vi "报告-报警采集.vi"   [LabVIEW 2015]
uses:
  Global control/global-1.vi
  Global control/global-Report.vi
  Global control/global-2.vi
  Global control/global-opc.vi
types:
  T1 = cluster{"Host交流故障":bool, "Host交流缺相":bool, "Host交流失电":bool, "01#JLCL交流故障":bool, "01#JLCL交流缺相":bool, "01#JLCL交流失电":bool, "02#JLCL交流故障":bool, "02#JLCL交流缺相":bool, "02#JLCL交流失电":bool, "备用1":bool, "备用2":bool, "备用3":bool, "备用4":bool, "备用5":bool, "备用6":bool, " 备用7":bool}
  T2 = cluster{"09#电源模块故障":bool, "10#电源模块故障":bool, "11#电源模块故障":bool, "12#电源模块故障":bool, "13#电源模块故障":bool, "14#电源模块故障":bool, "15#电源模块故障":bool, "16#电源模块故障":bool, "01#电源模块故障":bool, "02#电源模块故障":bool, "03#电源模块故障":bool, "04#电源模块故障":bool, "05#电源模块故障":bool, "06#电源模块故障":bool, "07#电源模块故障":bool, " 08#电源模块故障":bool}
  T3 = cluster{"09#模块通信故障":bool, "10#模块通信故障":bool, "11#模块通信故障":bool, "12#模块通信故障":bool, "13#模块通信故障":bool, "14#模块通信故障":bool, "15#模块通信故障":bool, "16#模块通信故障":bool, "01#模块通信故障":bool, "02#模块通信故障":bool, "03#模块通信故障":bool, "04#模块通信故障":bool, "05#模块通信故障":bool, "06#模块通信故障":bool, "07#模块通信故障":bool, "08#模块通信故障":bool}
  T4 = cluster{"母线过压":bool, "母线欠压":bool, "母线绝缘异常":bool, "母线绝缘预警":bool, "母线绝缘压差故障":bool, "母线交流串入故障":bool, "备用5":bool, " 备用6":bool, "电池组过压":bool, "电池组欠压":bool, "电池组过温":bool, "单体电池故障":bool, "备用1":bool, "备用2":bool, "备用3":bool, " 备用4":bool}
  T5 = cluster{"合母输出3#告警":bool, "合母输出4#告警":bool, "合母输出5#告警":bool, "合母输出6#告警":bool, "13#开关状态":bool, "14#开关状态":bool, "15#开关状态":bool, "16#开关状态":bool, "控母输出1#告警":bool, "控母输出2#告警":bool, "控母输出3#告警":bool, "控母输出4#告警":bool, "控母输出5#告警":bool, "控母输出6#告警":bool, "合母输出1#告警":bool, "合母输出2#告警":bool}
  T6 = cluster{"动作报告1":bool, "动作报告2":bool, "动作报告3":bool, "动作报告4":bool, "动作报告5":bool, "动作报告6":bool, "动作报告7":bool, "动作报告8":bool, "动作报告9":bool, "动作报告10":bool, "动作报告11":bool, "动作报告12":bool, "动作报告13":bool, "动作报告14":bool, "动作报告15":bool, "动作报告16":bool, "重合闸成功":bool, "线路测试失败":bool, "重合闸失败":bool, "手动合闸失败":bool, "一次重合":bool, "二次重合":bool, "三次重合":bool, "四次重合":bool, "失灵保护跳闸":bool, "失灵保护重跳":bool}
  T7 = cluster{"动作信号":bool, "异常告警":bool, "断路器合闸位置":bool, "隔离开关合闸位置":bool, "远方就地（1就地）":bool, "扩展板异常告警":bool, "虚遥信7":bool, "虚遥信8":bool, "虚遥信9":bool, "虚遥信10":bool, "虚遥信11":bool, "虚遥信12":bool, "虚遥信13":bool, "虚遥信14":bool, "虚遥信15":bool, "虚遥信16":bool}
  T8 = cluster{"直接合闸":bool, "分闸复位":bool, "带测合闸":bool, "MCB故障":bool, "断路器合闸反馈信号":bool, "ED储能":bool, "应急分闸":bool, "断路器分闸反馈信号":bool, "远程控制":bool, "就地控制":bool, "试验位置":bool, "工作位置":bool, "带测接触器":bool, "本站框架":bool, "邻站过流":bool, "邻站框架":bool}
  T9 = cluster{"toHMI正常运行":bool, "toHMI异常跳闸":bool, "toHMI远程":bool, "toHMI模拟中压合闸—按钮":bool, "toHMI负极柜故障报警":bool, "toHMI正极柜故障报警":bool, "toHMI馈线柜故障报警":bool, "toHMI上网柜故障报警":bool, "toHMI整流柜故障报警":bool, "toHMI压敏快熔故障":bool, "toHMI整流柜跳闸":bool, "toHMI整流柜合闸—状态":bool, "直流电流输出":u32, "直流220V电压输出":u32, "380电压输入":u32, "模拟中压合闸控制":bool, "toHMI本地":bool}
  T10 = cluster{"toHMI正常运行":bool, "toHMI设备准备好":bool, "toHMI设备异常":bool, "toHMI刀开关合—状态":bool, "toHMI刀开关分—状态":bool, "toHMI刀开关合按钮":bool, "toHMI刀开关分按钮":bool, "toHMI复位按钮":bool, "toHMI远程":bool, "toHMI本地":bool, "toHMI刀闸合—动作":bool, "toHMI刀闸分—动作":bool, "刀开关合闸控制":bool, "刀开关分闸控制":bool, "故障复位控制":bool}
  T11 = cluster{"toHMI正常运行":bool, "toHMI设备准备好":bool, "toHMI设备异常":bool, "toHMI高断分—状态":bool, "toHMI高断合—状态":bool, "toHMI继保故障信号":bool, "toHMI远方":bool, "toHMI本地":bool, "toHMI旁路合闸—按钮":bool, "toHMI旁路分闸—按钮":bool, "toHMI允许高断合闸—状态":bool, "toHMI旁路合分闸—状态":bool, "1500V电压输出":u32, "高断储能控制":bool, "旁路合闸控制":bool, "旁路分闸控制":bool}
  T12 = cluster{"toHMI正常运行":bool, "toHMI设备准备好":bool, "toHMI设备异常":bool, "toHMI刀开关分—状态":bool, "toHMI刀开关合—状态":bool, "toHMI框架电流故障":bool, "toHMI框架电压故障":bool, "toHMII段电压故障":bool, "toHMIII段电压故障":bool, "toHMI装置故障":bool, "toHMIMCB故障":bool, "toHMI刀开关合—完成":bool, "toHMI复位按钮":bool, "toHMI远程":bool, "toHMI本地":bool, "模拟电流框架故障控制":bool, "模拟电压框架故障控制":bool, "模拟I段电压故障控制":bool, "模拟II段电压故障控制":bool, "故障复位控制":bool}
  T13 = cluster{"toHMI刀开关合—状态":bool, "toHMI刀开关分—状态":bool, "toHMI刀开关合按钮":bool, "toHMI刀开关分按钮":bool, "toHMI远程":bool, "toHMI本地":bool, "toHMI正常运行":bool, "toHMI设备准备好":bool, "toHMI设备异常":bool, "toHMI刀闸合—动作":bool, "toHMI刀闸分—动作":bool, "toHMI接触轨有压":bool, "刀开关合闸控制":bool, "刀开关分闸控制":bool}
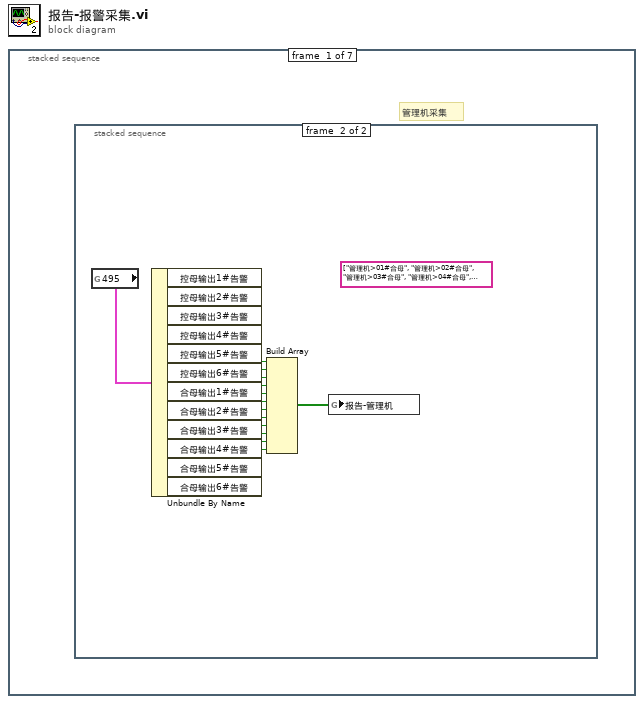
[diagram p0: block diagram]
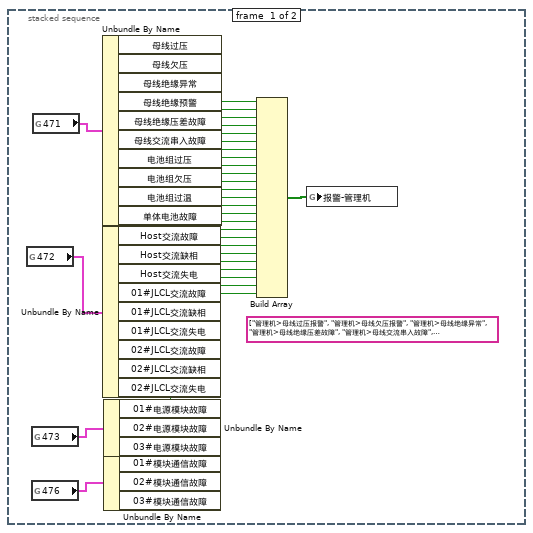
[diagram p2: hidden frame]
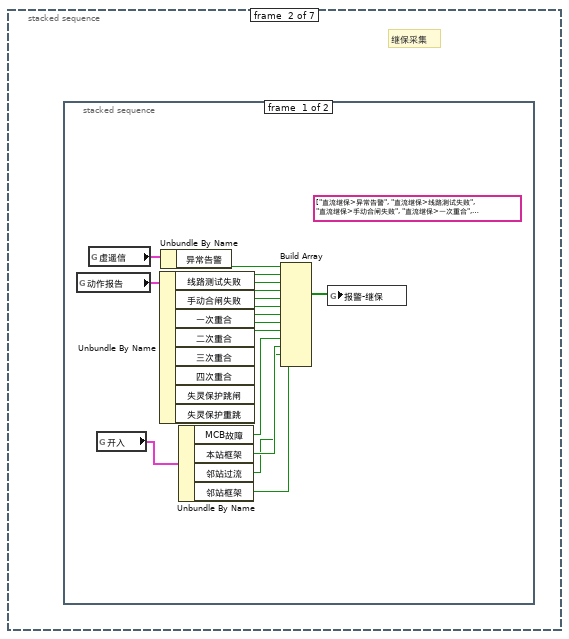
[diagram p3: hidden frame]
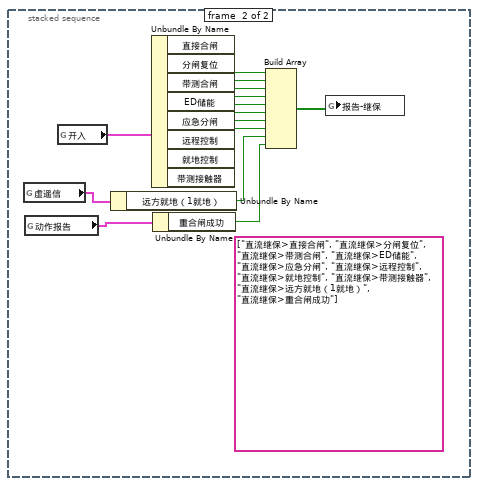
[diagram p4: hidden frame]
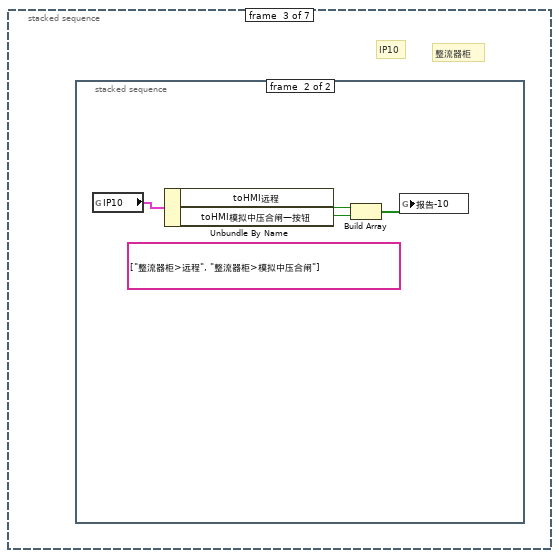
[diagram p5: hidden frame]
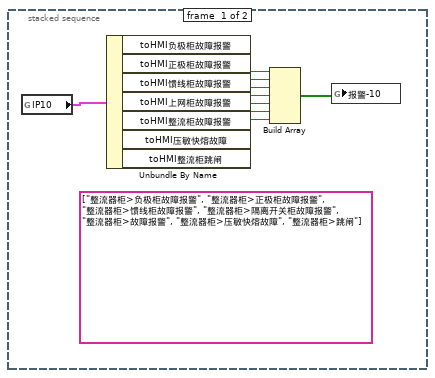
[diagram p6: hidden frame]
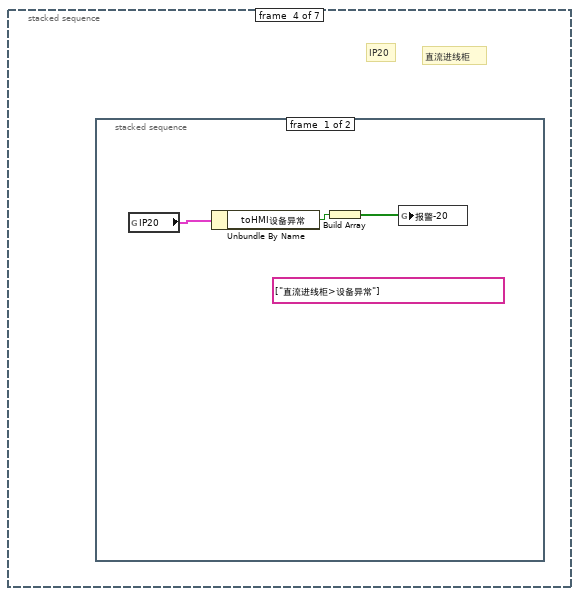
[diagram p7: hidden frame]
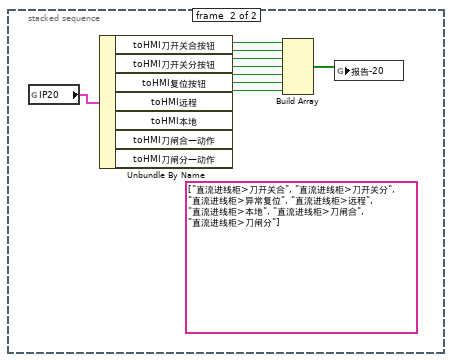
[diagram p8: hidden frame]
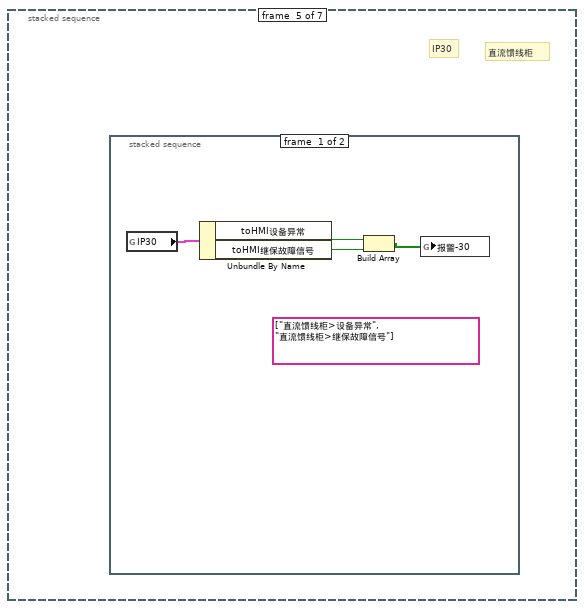
[diagram p9: hidden frame]
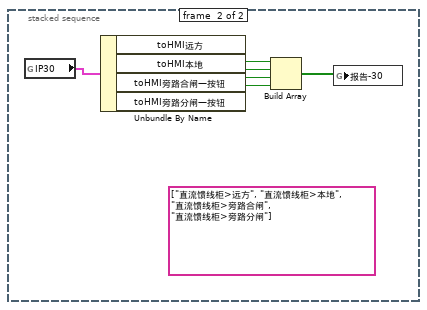
[diagram p10: hidden frame]
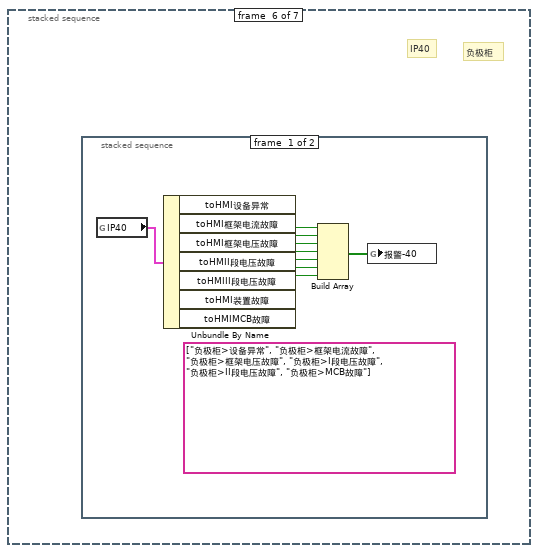
[diagram p11: hidden frame]
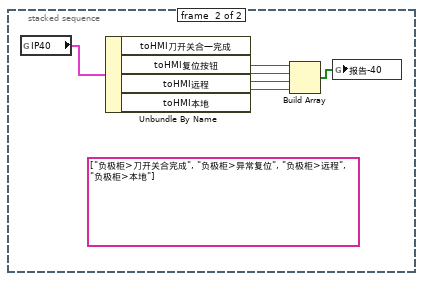
[diagram p12: hidden frame]
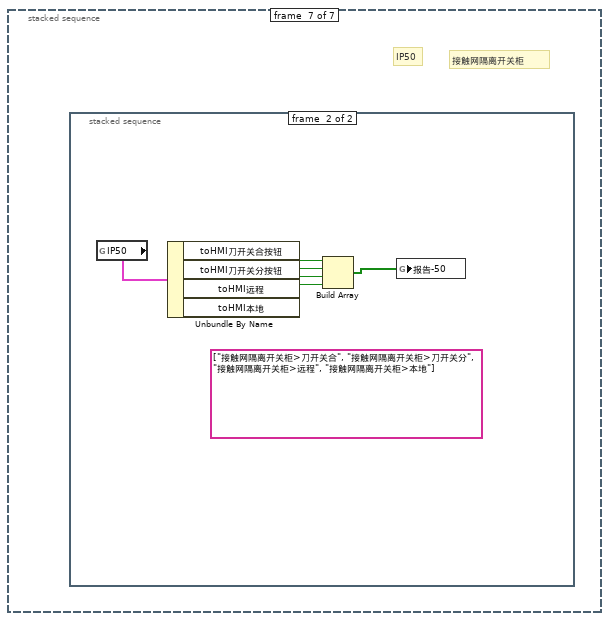
[diagram p13: hidden frame]
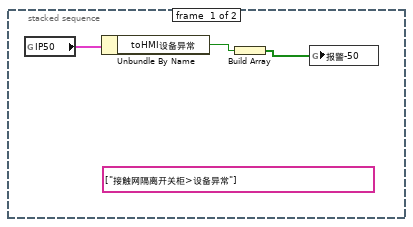
[diagram p14: hidden frame]
diagram:
  n1 = stacked-sequence {
    frame #0 {
      # "管理机采集"
      n2 = stacked-sequence {
        frame #0 {
          (unwired) string[] ["管理机>母线过压报警", "管理机>母线欠压报警", "管理机>母线绝缘异常", "管理机>母线绝缘压差故障", "管理机>母线交流串入故障", "管理机>电池组过压", "管理机>电池组欠压", "管理机>电池组过温", "管理机>单体电池故障", "管理机>Host交流故障", "管理机>Host交流缺相", "管理机>Host交流失电", "管理机>01#JLCL交流故障", "管理机>01#JLCL交流缺相", "管理机>01#JLCL交流失电", "管理机>02#JLCL交流故障", "管理机>02#JLCL交流缺相", "管理机>02#JLCL交流失电", "管理机>01#电源模块故障", "管理机>02#电源模块故障", "管理机>03#电源模块故障", "管理机>01##模块通信故障", "管理机>02##模块通信故障", "管理机>03##模块通信故障"]
          n3 = global read "global-1.vi" "472"() -> (w29:T1)
          n4 = global read "global-1.vi" "473"() -> (w28:T2)
          n5 = global read "global-1.vi" "476"() -> (w27:T3)
          n6 = global read "global-1.vi" "471"() -> (w30:T4)
          n7 = Unbundle By Name(w30) -> ("母线过压"=w26:bool, "母线欠压"=w25:bool, "母线绝缘异常"=w24:bool, "母线绝缘预警"=w23:bool, "母线绝缘压差故障"=w22:bool, "母线交流串入故障"=w21:bool, "电池组过压"=w20:bool, "电池组欠压"=w19:bool, "电池组过温"=w18:bool, "单体电池故障"=w17:bool)
          n8 = Unbundle By Name(w29) -> ("Host交流故障"=w16:bool, "Host交流缺相"=w15:bool, "Host交流失电"=w14:bool, "01#JLCL交流故障"=w13:bool, "01#JLCL交流缺相"=w12:bool, "01#JLCL交流失电"=w11:bool, "02#JLCL交流故障"=w10:bool, "02#JLCL交流缺相"=w9:bool, "02#JLCL交流失电"=w8:bool)
          n9 = Unbundle By Name(w28) -> ("01#电源模块故障"=w7:bool, "02#电源模块故障"=w6:bool, "03#电源模块故障"=w5:bool)
          n10 = Unbundle By Name(w27) -> ("01#模块通信故障"=w4:bool, "02#模块通信故障"=w3:bool, "03#模块通信故障"=w2:bool)
          n11 = Build Array(w26, w25, w24, w23, w22, w21, w20, w19, w18, w17, w16, w15, w14, w13, w12, w11, w10, w9, w8, w7, w6, w5, w4, w3, w2) -> (w1:bool[])
          n12 = global write "global-Report.vi" "报警-管理机"(w1) -> ()
        }
        frame #1 {
          (unwired) string[] ["管理机>01#合母", "管理机>02#合母", "管理机>03#合母", "管理机>04#合母", "管理机>05#合母", "管理机>06#合母", "管理机>01#控母", "管理机>02#控母", "管理机>03#控母", "管理机>04#控母", "管理机>05#控母", "管理机>06#控母"]
          n13 = global read "global-1.vi" "495"() -> (w44:T5)
          n14 = Unbundle By Name(w44) -> ("控母输出1#告警"=w43:bool, "控母输出2#告警"=w42:bool, "控母输出3#告警"=w41:bool, "控母输出4#告警"=w40:bool, "控母输出5#告警"=w39:bool, "控母输出6#告警"=w38:bool, "合母输出1#告警"=w37:bool, "合母输出2#告警"=w36:bool, "合母输出3#告警"=w35:bool, "合母输出4#告警"=w34:bool, "合母输出5#告警"=w33:bool, "合母输出6#告警"=w32:bool)
          n15 = Build Array(w43, w42, w41, w40, w39, w38, w37, w36, w35, w34, w33, w32) -> (w31:bool[])
          n16 = global write "global-Report.vi" "报告-管理机"(w31) -> ()
        }
      }
    }
    frame #1 {
      # "继保采集"
      n17 = stacked-sequence {
        frame #0 {
          (unwired) string[] ["直流继保>异常告警", "直流继保>线路测试失败", "直流继保>手动合闸失败", "直流继保>一次重合", "直流继保>二次重合", "直流继保>三次重合", "直流继保>四次重合", "直流继保>失灵保护跳闸", "直流继保>失灵保护重跳", "直流继保>MCB故障", "直流继保>本站框架", "直流继保>邻站过流", "直流继保>邻站框架"]
          n18 = global read "global-2.vi" "动作报告"() -> (w60:T6)
          n19 = global read "global-2.vi" "虚遥信"() -> (w61:T7)
          n20 = global read "global-2.vi" "开入"() -> (w49:T8)
          n21 = Unbundle By Name(w60) -> ("线路测试失败"=w58:bool, "手动合闸失败"=w57:bool, "一次重合"=w56:bool, "二次重合"=w55:bool, "三次重合"=w54:bool, "四次重合"=w53:bool, "失灵保护跳闸"=w52:bool, "失灵保护重跳"=w51:bool)
          n22 = Unbundle By Name(w61) -> ("异常告警"=w59:bool)
          n23 = Unbundle By Name(w49) -> ("MCB故障"=w48:bool, "本站框架"=w47:bool, "邻站过流"=w46:bool, "邻站框架"=w45:bool)
          n24 = Build Array(w59, w58, w57, w56, w55, w54, w53, w52, w51, w48, w47, w46, w45) -> (w50:bool[])
          n25 = global write "global-Report.vi" "报警-继保"(w50) -> ()
        }
        frame #1 {
          (unwired) string[] ["直流继保>直接合闸", "直流继保>分闸复位", "直流继保>带测合闸", "直流继保>ED储能", "直流继保>应急分闸", "直流继保>远程控制", "直流继保>就地控制", "直流继保>带测接触器", "直流继保>远方就地（1就地）", "直流继保>重合闸成功"]
          n26 = global read "global-2.vi" "虚遥信"() -> (w74:T7)
          n27 = global read "global-2.vi" "动作报告"() -> (w73:T6)
          n28 = global read "global-2.vi" "开入"() -> (w75:T8)
          n29 = Unbundle By Name(w74) -> ("远方就地（1就地）"=w64:bool)
          n30 = Unbundle By Name(w75) -> ("直接合闸"=w72:bool, "分闸复位"=w71:bool, "带测合闸"=w70:bool, "ED储能"=w69:bool, "应急分闸"=w68:bool, "远程控制"=w67:bool, "就地控制"=w66:bool, "带测接触器"=w65:bool)
          n31 = Unbundle By Name(w73) -> ("重合闸成功"=w63:bool)
          n32 = Build Array(w72, w71, w70, w69, w68, w67, w66, w65, w64, w63) -> (w62:bool[])
          n33 = global write "global-Report.vi" "报告-继保"(w62) -> ()
        }
      }
    }
    frame #2 {
      # "整流器柜"
      # "IP10"
      n34 = stacked-sequence {
        frame #0 {
          (unwired) string[] ["整流器柜>负极柜故障报警", "整流器柜>正极柜故障报警", "整流器柜>馈线柜故障报警", "整流器柜>隔离开关柜故障报警", "整流器柜>故障报警", "整流器柜>压敏快熔故障", "整流器柜>跳闸"]
          n35 = global read "global-opc.vi" "IP10"() -> (w84:T9)
          n36 = Unbundle By Name(w84) -> ("toHMI负极柜故障报警"=w83:bool, "toHMI正极柜故障报警"=w82:bool, "toHMI馈线柜故障报警"=w81:bool, "toHMI上网柜故障报警"=w80:bool, "toHMI整流柜故障报警"=w79:bool, "toHMI压敏快熔故障"=w78:bool, "toHMI整流柜跳闸"=w77:bool)
          n37 = Build Array(w83, w82, w81, w80, w79, w78, w77) -> (w76:bool[])
          n38 = global write "global-Report.vi" "报警-10"(w76) -> ()
        }
        frame #1 {
          (unwired) string[] ["整流器柜>远程", "整流器柜>模拟中压合闸"]
          n39 = global read "global-opc.vi" "IP10"() -> (w88:T9)
          n40 = Unbundle By Name(w88) -> ("toHMI远程"=w87:bool, "toHMI模拟中压合闸—按钮"=w86:bool)
          n41 = Build Array(w87, w86) -> (w85:bool[])
          n42 = global write "global-Report.vi" "报告-10"(w85) -> ()
        }
      }
    }
    frame #3 {
      # "直流进线柜"
      # "IP20"
      n43 = stacked-sequence {
        frame #0 {
          (unwired) string[] ["直流进线柜>设备异常"]
          n44 = global read "global-opc.vi" "IP20"() -> (w91:T10)
          n45 = Unbundle By Name(w91) -> ("toHMI设备异常"=w89:bool)
          n46 = Build Array(w89) -> (w90:bool[])
          n47 = global write "global-Report.vi" "报警-20"(w90) -> ()
        }
        frame #1 {
          (unwired) string[] ["直流进线柜>刀开关合", "直流进线柜>刀开关分", "直流进线柜>异常复位", "直流进线柜>远程", "直流进线柜>本地", "直流进线柜>刀闸合", "直流进线柜>刀闸分"]
          n48 = global read "global-opc.vi" "IP20"() -> (w100:T10)
          n49 = Unbundle By Name(w100) -> ("toHMI刀开关合按钮"=w99:bool, "toHMI刀开关分按钮"=w98:bool, "toHMI复位按钮"=w97:bool, "toHMI远程"=w96:bool, "toHMI本地"=w95:bool, "toHMI刀闸合—动作"=w94:bool, "toHMI刀闸分—动作"=w93:bool)
          n50 = Build Array(w99, w98, w97, w96, w95, w94, w93) -> (w92:bool[])
          n51 = global write "global-Report.vi" "报告-20"(w92) -> ()
        }
      }
    }
    frame #4 {
      # "直流馈线柜"
      # "IP30"
      n52 = stacked-sequence {
        frame #0 {
          (unwired) string[] ["直流馈线柜>设备异常", "直流馈线柜>继保故障信号"]
          n53 = global read "global-opc.vi" "IP30"() -> (w104:T11)
          n54 = Unbundle By Name(w104) -> ("toHMI设备异常"=w103:bool, "toHMI继保故障信号"=w102:bool)
          n55 = Build Array(w103, w102) -> (w101:bool[])
          n56 = global write "global-Report.vi" "报警-30"(w101) -> ()
        }
        frame #1 {
          (unwired) string[] ["直流馈线柜>远方", "直流馈线柜>本地", "直流馈线柜>旁路合闸", "直流馈线柜>旁路分闸"]
          n57 = global read "global-opc.vi" "IP30"() -> (w110:T11)
          n58 = Unbundle By Name(w110) -> ("toHMI远方"=w109:bool, "toHMI本地"=w108:bool, "toHMI旁路合闸—按钮"=w107:bool, "toHMI旁路分闸—按钮"=w106:bool)
          n59 = Build Array(w109, w108, w107, w106) -> (w105:bool[])
          n60 = global write "global-Report.vi" "报告-30"(w105) -> ()
        }
      }
    }
    frame #5 {
      # "负极柜"
      # "IP40"
      n61 = stacked-sequence {
        frame #0 {
          (unwired) string[] ["负极柜>设备异常", "负极柜>框架电流故障", "负极柜>框架电压故障", "负极柜>I段电压故障", "负极柜>II段电压故障", "负极柜>MCB故障"]
          n62 = global read "global-opc.vi" "IP40"() -> (w119:T12)
          n63 = Unbundle By Name(w119) -> ("toHMI设备异常"=w118:bool, "toHMI框架电流故障"=w117:bool, "toHMI框架电压故障"=w116:bool, "toHMII段电压故障"=w115:bool, "toHMIII段电压故障"=w114:bool, "toHMI装置故障"=w113:bool, "toHMIMCB故障"=w112:bool)
          n64 = Build Array(w118, w117, w116, w115, w114, w113, w112) -> (w111:bool[])
          n65 = global write "global-Report.vi" "报警-40"(w111) -> ()
        }
        frame #1 {
          (unwired) string[] ["负极柜>刀开关合完成", "负极柜>异常复位", "负极柜>远程", "负极柜>本地"]
          n66 = global read "global-opc.vi" "IP40"() -> (w125:T12)
          n67 = Unbundle By Name(w125) -> ("toHMI刀开关合—完成"=w124:bool, "toHMI复位按钮"=w123:bool, "toHMI远程"=w122:bool, "toHMI本地"=w121:bool)
          n68 = Build Array(w124, w123, w122, w121) -> (w120:bool[])
          n69 = global write "global-Report.vi" "报告-40"(w120) -> ()
        }
      }
    }
    frame #6 {
      # "接触网隔离开关柜"
      # "IP50"
      n70 = stacked-sequence {
        frame #0 {
          (unwired) string[] ["接触网隔离开关柜>设备异常"]
          n71 = global read "global-opc.vi" "IP50"() -> (w128:T13)
          n72 = Unbundle By Name(w128) -> ("toHMI设备异常"=w127:bool)
          n73 = Build Array(w127) -> (w126:bool[])
          n74 = global write "global-Report.vi" "报警-50"(w126) -> ()
        }
        frame #1 {
          (unwired) string[] ["接触网隔离开关柜>刀开关合", "接触网隔离开关柜>刀开关分", "接触网隔离开关柜>远程", "接触网隔离开关柜>本地"]
          n75 = global read "global-opc.vi" "IP50"() -> (w134:T13)
          n76 = Unbundle By Name(w134) -> ("toHMI刀开关合按钮"=w133:bool, "toHMI刀开关分按钮"=w132:bool, "toHMI远程"=w131:bool, "toHMI本地"=w130:bool)
          n77 = Build Array(w133, w132, w131, w130) -> (w129:bool[])
          n78 = global write "global-Report.vi" "报告-50"(w129) -> ()
        }
      }
    }
  }
